vi "export spectra.vi"(10 "Sample cluster":T4={"General description"="", "Sample setup"={"integration time"=0.5, "rinse time"=10.0, "sample time"=10.0, "sample type"=0}, "Absorbance"=[], "Analyst"="", "Sample descriptions"=[], "good data"=[]} {"Absorbance" format="%.2e"; "Sample setup"."sample type" items=["Sample Cuvet", "Sipper Cell", "No Dialog"]; "Sample setup"."sample time" min=0.0 max=100.0 step=1.0 format="%.1f"; "Sample setup"."rinse time" min=0.0 max=100.0 step=1.0 format="%.1f"; "Sample setup"."integration time" format="%.1f"}, 11 "standard cluster":T2={"Description"="", "Setup"={"integration time"=0.5, "rinse time"=10.0, "sample time"=10.0, "sample type"=0}, "Concentrations"=[], "Absorbance"=[], "Analyst"="", "Concentration units"="", "Good"=[]} {"Absorbance" format="%.2e"; "Concentrations" format="%.3e"; "Setup"."sample type" items=["Sample Cuvet", "Sipper Cell", "No Dialog"]; "Setup"."sample time" min=0.0 max=100.0 step=1.0 format="%.1f"; "Setup"."rinse time" min=0.0 max=100.0 step=1.0 format="%.1f"; "Setup"."integration time" format="%.1f"}) -> ()   [LabVIEW 2015]
uses:
  sample cluster.ctl
  settings.ctl
  standard cluster.ctl
  <vilib>/Analysis/1siggen.llb/Ramp Pattern by Samples.vi
  <vilib>/Utility/file.llb/Write To Spreadsheet File (DBL).vi
  <vilib>/Utility/file.llb/Write Delimited Spreadsheet (DBL).vi
  <vilib>/Utility/file.llb/Write Delimited Spreadsheet (string).vi
  <vilib>/Analysis/NI_AALBase.lvlib
panel:
  in  "stop":bool
  in  "state":T1
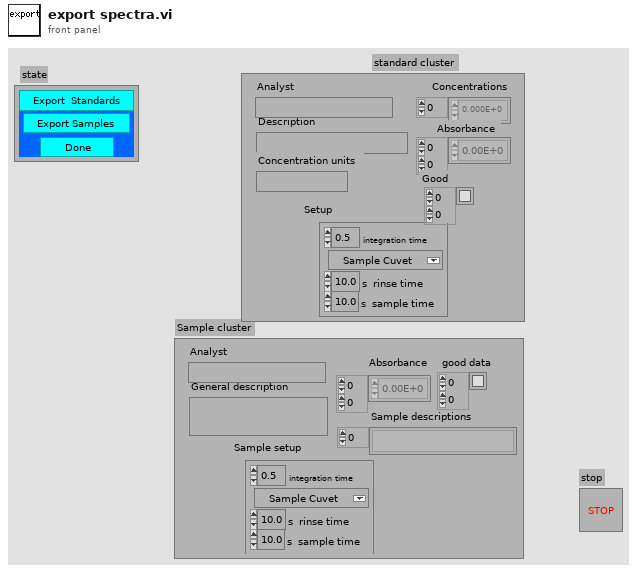
[diagram p1: front panel]
types:
  T1 = cluster{"Load Standards":bool, "Load Unknowns":bool, "Quit":bool}
  T2 = typedef "standard cluster.ctl" = cluster{"Description":string, "Setup":T3, "Concentrations":dbl[], "Absorbance":dbl[][], "Analyst":string, "Concentration units":string, "Good":bool[][]}
  T3 = typedef "settings.ctl" = cluster{"integration time":sgl, "rinse time":dbl[unit], "sample time":dbl[unit], "sample type":u16}
  T4 = typedef "sample cluster.ctl" = cluster{"General description":string, "Sample setup":T3, "Absorbance":dbl[][], "Analyst":string, "Sample descriptions":string[], "good data":bool[][]}
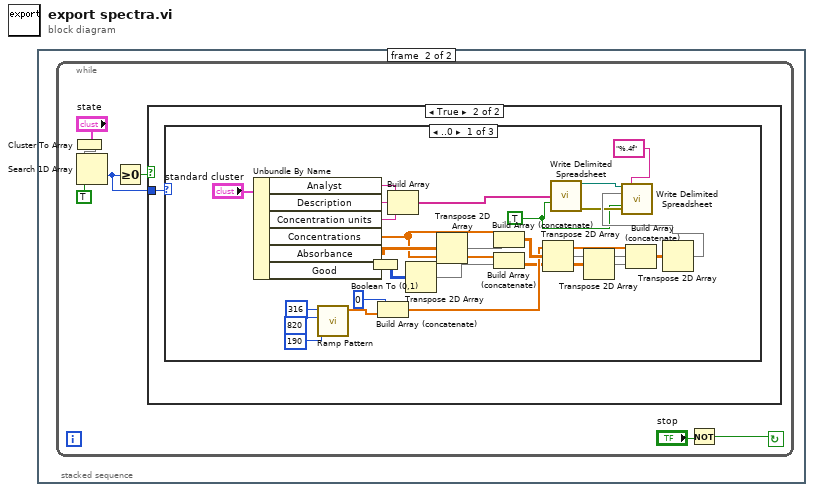
[diagram p0: block diagram]
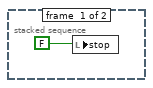
[diagram p2: hidden frame]
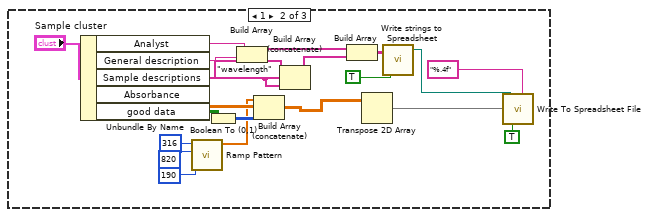
[diagram p4: hidden frame]
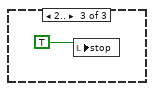
[diagram p5: hidden frame]
diagram:
  n1 = stacked-sequence {
    frame #0 {
      n2 = local write "stop"(FALSE) -> ()
    }
    frame #1 {
      n3 = while {
        stop <- w2 continue-if-true
        n4 = Cluster To Array(cluster="state") -> (array=w4:bool[])
        n5 = Search 1D Array(1D array=w4, element=TRUE) -> (index of element=w7:i32)  [unwired: 1 in]
        n6 = Greater Or Equal To 0?(x=w7) -> (x >= 0?=w6:bool)
        n7 = case shown="True" w6 {
          tunnel: w7 -> [_ w9]
          frame False {
          }
          frame True {
            n8 = case shown="..0" w9 {
              frame ..0 {
                w11 = TRUE ("append to file? (new file:F)")
                n9 = Unbundle By Name("standard cluster") -> ("Analyst"=w17:string, "Description"=w18:string, "Concentration units"=w19:string, "Concentrations"=w26:dbl[], "Absorbance"=w29:dbl[][], "Good"=w23:bool[][])
                n10 = call-poly <vilib>:"Ramp Pattern.vi"("start"=190, "end"=820, "samples"=316) -> ("Ramp Pattern"=w24:dbl[])  [unwired: 7 in, 1 out]
                n11 = Boolean To (0,1)(Boolean=w23) -> (0, 1=w30:i16[][])
                n12 = Build Array (concatenate)(0, w24) -> (w33:dbl[])
                n13 = Build Array(w17, w18, w19) -> (w10:string[])
                n14 = Transpose 2D Array(2D array=w30) -> (transposed array=w32:i16[][])
                n15 = Transpose 2D Array(2D array=w29) -> (transposed array=w31:dbl[][])
                n16 = Build Array (concatenate)(w26, w31) -> (w34:dbl[][])
                n17 = Build Array (concatenate)(w26, w32) -> (w27:dbl[][])
                n18 = Transpose 2D Array(2D array=w34) -> (transposed array=w35:dbl[][])
                n19 = call-poly <vilib>:"Write Delimited Spreadsheet.vi"("1D data"=w10, "append to file? (F)"=w11) -> ("new file path (Not A Path if cancelled)"=w13:path, "error out"=w12:errorcluster)  [unwired: 12 in]
                n20 = Transpose 2D Array(2D array=w27) -> (transposed array=w36:dbl[][])
                n21 = Build Array (concatenate)(w33, w35, w36) -> (w28:dbl[][])
                n22 = Transpose 2D Array(2D array=w28) -> (transposed array=w14:dbl[][])
                n23 = call-poly <vilib>:"Write Delimited Spreadsheet.vi"("file path (dialog if empty)"=w13, "format (%.3f)"="%.4f", "2D data"=w14, "append to file? (F)"=w11, "error in (no error)"=w12) -> ()  [unwired: 9 in, 2 out]
              }
              frame 1 {
                n24 = Unbundle By Name("Sample cluster") -> ("Analyst"=w46:string, "General description"=w47:string, "Sample descriptions"=w39:string[], "Absorbance"=w53:dbl[][], "good data"=w52:bool[][])
                n25 = call-poly <vilib>:"Ramp Pattern.vi"("start"=190, "end"=820, "samples"=316) -> ("Ramp Pattern"=w41:dbl[])  [unwired: 7 in, 1 out]
                n26 = Boolean To (0,1)(Boolean=w52) -> (0, 1=w54:i16[][])
                n27 = Build Array(w46, w47) -> (w48:string[])
                n28 = Build Array (concatenate)(w41, w53, w54) -> (w40:dbl[][])
                n29 = Build Array (concatenate)("wavelength", w39, w39) -> (w51:string[])
                n30 = Build Array(w48, w51) -> (w49:string[][])
                n31 = Transpose 2D Array(2D array=w40) -> (transposed array=w38:dbl[][])
                n32 = call "Write strings to Spreadsheet"("append to file? (new file:F)"=TRUE, "2D data"=w49) -> ("new file path (Not A Path if cancelled)"=w57:path)  [unwired: 6 in]
                n33 = call-poly <vilib>:"Write To Spreadsheet File.vi"("format (%.3f)"="%.4f", "append to file? (new file:F)"=TRUE, "2D data"=w38, "file path (dialog if empty)"=w57) -> ()  [unwired: 4 in, 1 out]
              }
              frame 2.. {
                n34 = local write "stop"(TRUE) -> ()
              }
            }
          }
        }
        n35 = Not(x="stop") -> (.not. x?=w2:bool)
      }
    }
  }
